vi "Controlword_ModeSpecific_PositionProfile.vi"(7 "Halt":bool, 8 "Relative?":bool, 9 "Change Immediately? (If False, will Blend)":bool, 10 "New Setpoint?":bool, 11 "ControlWord In":u16 format="%08b") -> (3 "ControlWord Out":u16 format="%08b")   [LabVIEW 2017, in "WordManipulationLibrary.lvlib"]
uses:
  WordManipulationLibrary.lvlib
  Bit Manipulation.lvlib
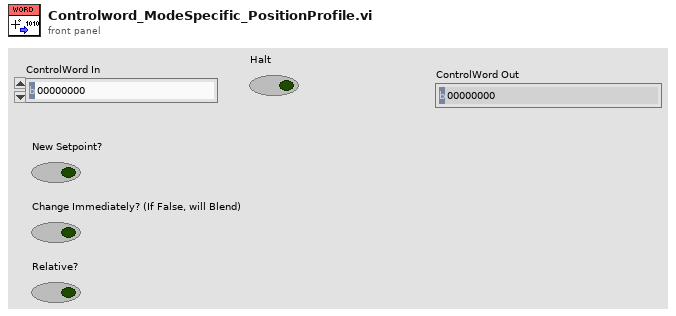
[diagram p1: front panel]
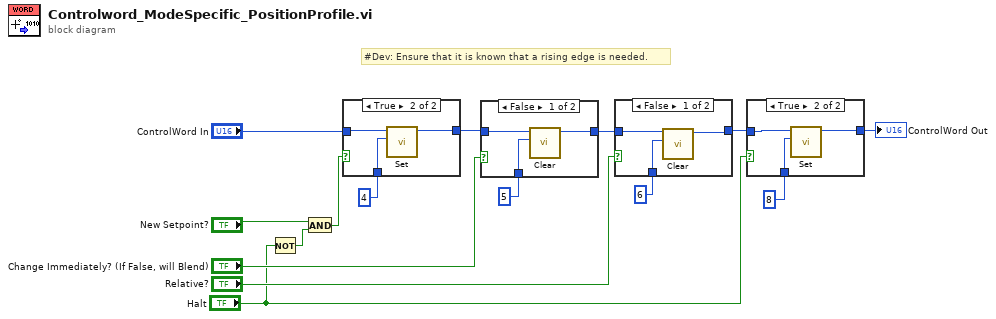
[diagram p0: block diagram]
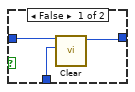
[diagram p2: hidden frame]
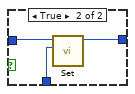
[diagram p3: hidden frame]
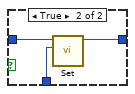
[diagram p4: hidden frame]
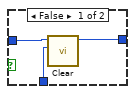
[diagram p5: hidden frame]
diagram:
  # "#Dev: Ensure that it is known that a rising edge is needed."
  n1 = Not(x="Halt") -> (.not. x?=w2:bool)
  n2 = And(x="New Setpoint?", y=w2) -> (x .and. y?=w1:bool)
  n3 = case shown="True" w1 {
    tunnel: "ControlWord In" -> [w18 w21]
    tunnel: [w17 w20] -> w14
    tunnel: u8 4 ("Bit to set") -> [w16 w19]
    frame False {
      n4 = call "Clear.vi"("Bit to clear"=w16, "Data_In"=w18) -> ("Data_Out"=w17:u16)  [unwired: 9 in]
    }
    frame True {
      n5 = call "Set.vi"("Bit to set"=w19, "Data_In"=w21) -> ("Data_Out"=w20:u16)  [unwired: 9 in]
    }
  }
  n6 = case shown="False" "Change Immediately? (If False, will Blend)" {
    tunnel: w14 -> [w23 w27]
    tunnel: [w24 w26] -> w13
    tunnel: u8 5 ("Bit to set") -> [w22 w25]
    frame False {
      n7 = call "Clear.vi"("Bit to clear"=w22, "Data_In"=w23) -> ("Data_Out"=w24:u16)  [unwired: 9 in]
    }
    frame True {
      n8 = call "Set.vi"("Bit to set"=w25, "Data_In"=w27) -> ("Data_Out"=w26:u16)  [unwired: 9 in]
    }
  }
  n9 = case shown="False" "Relative?" {
    tunnel: w13 -> [w30 w33]
    tunnel: [w29 w32] -> w9
    tunnel: u8 6 ("Bit to set") -> [w28 w31]
    frame False {
      n10 = call "Clear.vi"("Bit to clear"=w28, "Data_In"=w30) -> ("Data_Out"=w29:u16)  [unwired: 9 in]
    }
    frame True {
      n11 = call "Set.vi"("Bit to set"=w31, "Data_In"=w33) -> ("Data_Out"=w32:u16)  [unwired: 9 in]
    }
  }
  n12 = case shown="True" "Halt" {
    tunnel: w9 -> [w35 w38]
    tunnel: [w34 w39] -> w10
    tunnel: u8 8 ("Bit to set") -> [w36 w37]
    frame False {
      n13 = call "Clear.vi"("Bit to clear"=w36, "Data_In"=w35) -> ("Data_Out"=w34:u16)  [unwired: 9 in]
    }
    frame True {
      n14 = call "Set.vi"("Bit to set"=w37, "Data_In"=w38) -> ("Data_Out"=w39:u16)  [unwired: 9 in]
    }
  }
  "ControlWord Out" <- w10
